vi "Waveform Attribute, Get DBL.vi"(6 "error in":errorcluster, 8 "label":string, 9 "waveform":waveform(dbl)) -> (0 "error out":errorcluster, 1 "found":bool, 2 "value":dbl=nan format="%.3f", 3 "waveform dup":waveform(dbl)={"t0"=timestamp(0 s since 1904-01-01), "dt"=nan, "Y"=[]})   [LabVIEW 2010]
doc: "This function reads a double precision floating point value from a waveform attribute. If an error occurs, the value is set to NaN."
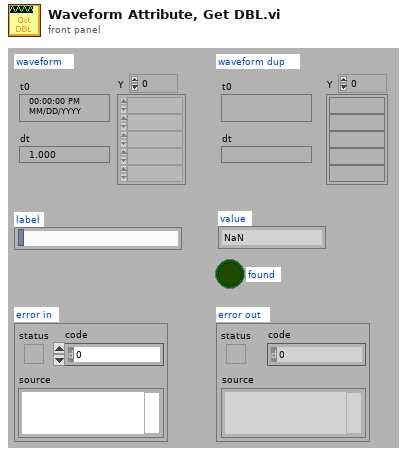
[diagram p1: front panel]
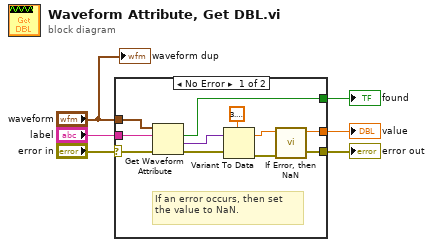
[diagram p0: block diagram]
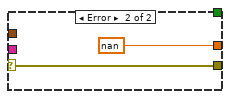
[diagram p2: hidden frame]
diagram:
  n1 = case shown="No Error" "error in" {
    selector: "error in" -> [w11 w19]
    tunnel: [w12 w19] -> w6
    tunnel: "waveform" -> [w17 _]
    tunnel: [w16 _] -> w4
    tunnel: "label" -> [w10 _]
    tunnel: [w7 nan ("value out1")] -> w1
    frame No Error {
      # "If an error occurs, then set the value to NaN."
      n2 = Get Waveform Attribute(4:w11, 6:w10, 7:w17) -> (0:w14:errorcluster, 1:w15:variant, 2:w16:bool)  [unwired: 1 in, 1 out]
      n3 = Variant To Data(error in=w14, Variant=w15, type=3.141592653589793) -> (error out=w13:errorcluster, data=w8:dbl)
      n4 = call "If Error, then NaN.vi"("error in (T)"=w13, "value1"=w8) -> ("error out"=w12:errorcluster, "value out1"=w7:dbl)  [unwired: 4 in, 2 out]
    }
    frame Error {
    }
  }
  "error out" <- w6
  "found" <- w4
  "value" <- w1
  "waveform dup" <- "waveform"
